vi "Is Open Status.vi"(8 "error in (no error)":errorcluster, 11 "TCPMessaging in":refnum<class "TCPMessaging.lvclass">) -> (0 "error out":errorcluster, 2 "Open":bool, 3 "TCPMessaging out":refnum<class "TCPMessaging.lvclass">)   [LabVIEW 2020, in "Vecto.lvlib" / "TCPMessaging.lvclass"]
uses:
  TCPMessaging.lvclass
  TCPMessaging.lvclass/TCPMessaging.ctl
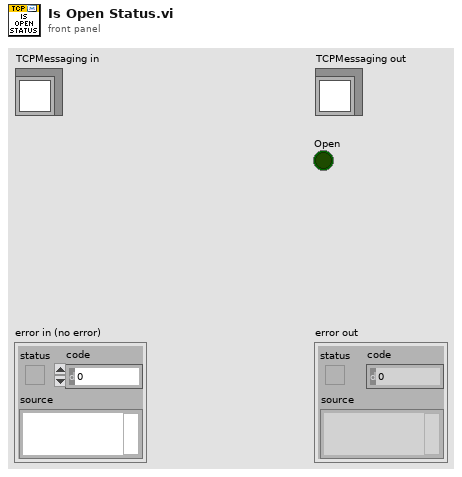
[diagram p1: front panel]
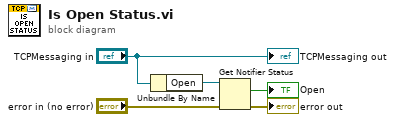
[diagram p0: block diagram]
diagram:
  n1 = Unbundle By Name("TCPMessaging in") -> ("Open"=w4:refnum<notifier>)
  n2 = Get Notifier Status(notifier=w4, error in (no error)="error in (no error)") -> (current notification=→"Open":bool, error out=→"error out":errorcluster)  [unwired: 3 out]
  "TCPMessaging out" <- "TCPMessaging in"
